vi "Dyanmixel Motor Read All Data From Motor(s).vi"() -> ()   [LabVIEW 2016]
doc: "This example shows how to collect all of the available data from a Dynamixel motor."
uses:
  <instrlib>/Dynamixel Motor/Public/Motor Operation/Low Level/Baud Setting.ctl
  <instrlib>/Dynamixel Motor/HAIOL/Dynamixel Motor.lvclass
  <instrlib>/Dynamixel Motor/HAIOL/VISA/Dynamixel Motor VISA.lvclass
  <instrlib>/Dynamixel Motor/Dynamixel Motor.lvlib
panel:
  in  "Force Baud Rate (True)":bool=TRUE
  in  "error in":errorcluster
  out "error out":errorcluster
  in  "Timeout (30 msec)":u32=30
  out "Motor Properties":string[][](table)
  in  "Motor ID List":u8[](array[numeric])
  in  "Baud rate (57600 bps)":T1=34 items=["1,000,000 bps"=1, "500,000 bps"=3, "400,000 bps"=4, "250,000 bps"=7, "200,000 bps"=9, "115200 bps"=16, "57600 bps"=34, "19200 bps"=103, "9600 bps"=207]
  in  "VISA resource name":refnum<visa-resource-name>
  # "(c) 2011  National Instruments.  ALL RIGHTS RESERVED."
  # "Input the motor IDs of all of the motors connected in the chain that you want to query.  Then run the VI."
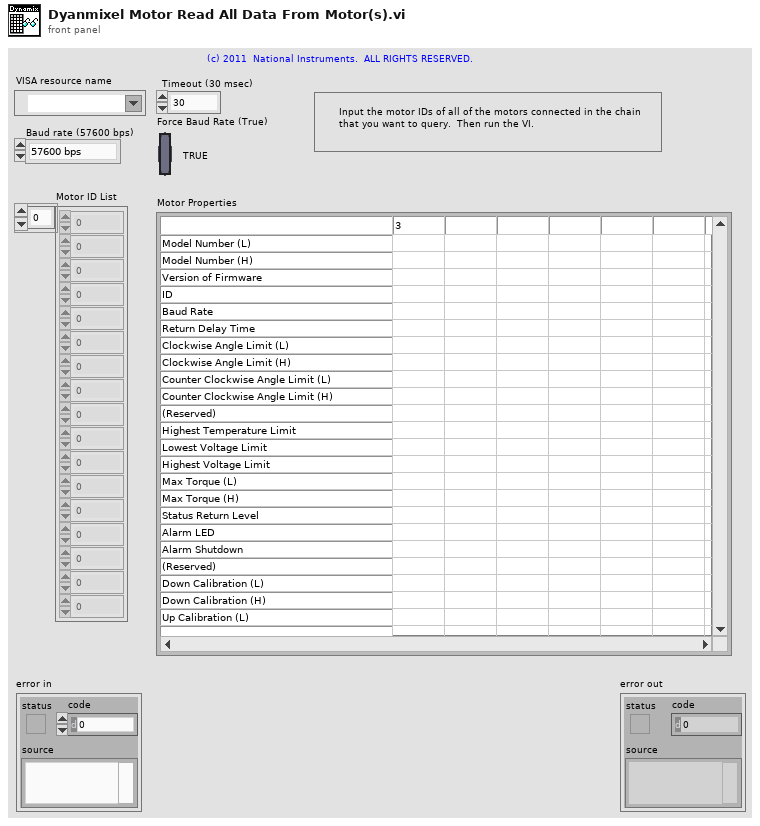
[diagram p1: front panel]
types:
  T1 = typedef "Dynamixel Motor.lvlib/Baud Setting.ctl" = u8
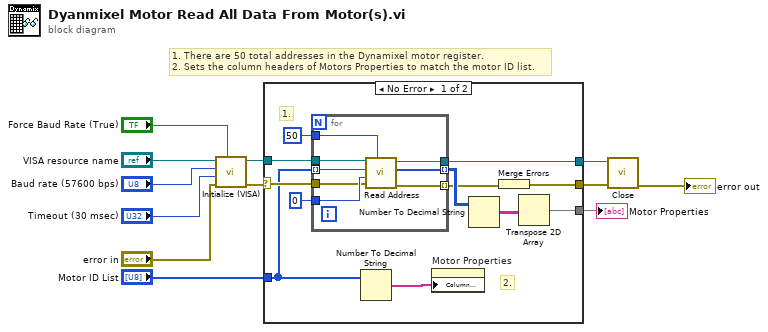
[diagram p0: block diagram]
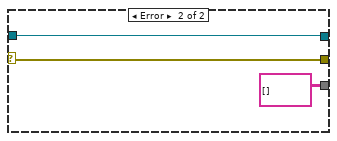
[diagram p2: hidden frame]
diagram:
  # "1. There are 50 total addresses in the Dynamixel motor register.\n2. Sets the column headers of Motors Properties to match the motor ID list."
  n1 = call <instrlib>:"Initialize (VISA).vi"("Force Baud Rate (True)"="Force Baud Rate (True)", "error in (no error)"="error in", "Timeout (30 msec)"="Timeout (30 msec)", "Baud rate (57600 bps)"="Baud rate (57600 bps)", "VISA resource name"="VISA resource name") -> ("error out"=w7:errorcluster, "Dynamixel Motor out"=w6:refnum<class "Dynamixel Motor.lvclass">)  [unwired: 5 in]
  n2 = case shown="No Error" w7 {
    selector: w7 -> [w22 w35]
    tunnel: w6 -> [w24 w34]
    tunnel: "Motor ID List" -> [w19 _]
    tunnel: [w15 w35] -> w2
    tunnel: [w14 w34] -> w3
    tunnel: [w13 string[][] []] -> w4
    frame No Error {
      # "2."
      # "1."
      n3 = for {
        tunnel: w24 -> [w32]
        tunnel: w19 -> [w31] mode=indexing
        tunnel: u8 0 ("Address number (0)") -> [w30]
        tunnel: w22 -> [w29]
        tunnel: u8 50 ("Number of Addresses to read (1)") -> [w28]
        tunnel: [w27] -> w14
        tunnel: [w26] -> w17 mode=indexing
        tunnel: [w25] -> w16 mode=indexing
        n4 = call-dynamic "Read Address.vi"("Number of Addresses to read (1)"=w28, "error in (no error)"=w29, "Address number (0)"=w30, "Motor ID (0)"=w31, "Dynamixel Motor in"=w32) -> ("error out"=w25:errorcluster, "Data Read"=w26:u8[], "Dynamixel Motor out"=w27:refnum<class "Dynamixel Motor.lvclass">)  [unwired: 3 in, 1 out]
      }
      n5 = Number To Decimal String(number=w19) -> (decimal integer string=w20:string[])  [unwired: 1 in]
      n6 = property on="Motor Properties" class="Tbl (strict)"("Column Headers[]"=w20) -> ()  [unwired: 2 in, 2 out]
      n7 = Number To Decimal String(number=w17) -> (decimal integer string=w18:string[][])  [unwired: 1 in]
      n8 = Merge Errors(w16) -> (w15:errorcluster)
      n9 = Transpose 2D Array(2D array=w18) -> (transposed array=w13:string[][])
    }
    frame Error {
    }
  }
  "Motor Properties" <- w4
  n10 = call-dynamic "Close.vi"("error in (no error)"=w2, "Dynamixel Motor in"=w3) -> ("error out"=→"error out":errorcluster)  [unwired: 9 in]
